vi "DevScripts_EnumToEnum-GLAttr.vi"() -> ()   [LabVIEW 2024]
uses:
  <vilib>/Utility/error.llb/Trim Whitespace One-Sided.vi
  SDL3/Video/GLAttr--enum.ctl
  SDL3/Video/Video.lvlib
panel:
  out "spreadsheet string":string
  out "Array":string[](array[string])
  in  "#Define list":string="    SDL_GL_RED_SIZE,                    /**< the minimum number of bits for the red channel of the color buffer; defaults to 3. */\n    SDL_GL_GREEN_SIZE,                  /**< the minimum number of bits for the green channel of the color buffer; defaults to 3. */\n    SDL_GL_BLUE_SIZE,                   /**< the minimum number of bits for the blue channel of the color buffer; defaults to 2. */\n    SDL_GL_ALPHA_SIZE,                  /**< the minimum number of bits for the alpha channel of the color buffer; defaults to 0. */\n    SDL_GL_BUFFER_SIZE,                 /**< the minimum number of bits for frame buffer size; defaults to 0. */\n    SDL_GL_DOUBLEBUFFER,                /**< whether the output is single or double buffered; defaults to double buffering on. */\n    SDL_GL_DEPTH_SIZE,                  /**< the minimum number of bits in the depth buffer; defaults to 16. */\n    SDL_GL_STENCIL_SIZE,                /**< the minimum number of bits in the stencil buffer; defaults to 0. */\n    SDL_GL_ACCUM_RED_SIZE,              /**< the minimum number of bits for the red channel of the accumulation buffer; defaults to 0. */\n    SDL_GL_ACCUM_GREEN_SIZE,            /**< the minimum number of bits for the green channel of the accumulation buffer; defaults to 0. */\n    SDL_GL_ACCUM_BLUE_SIZE,             /**< the minimum number of bits for the blue channel of the accumulation buffer; defaults to 0. */\n    SDL_GL_ACCUM_ALPHA_SIZE,            /**< the minimum number of bits for the alpha channel of the accumulation buffer; defaults to 0. */\n    SDL_GL_STEREO,                      /**< whether the output is stereo 3D; defaults to off. */\n    SDL_GL_MULTISAMPLEBUFFERS,          /**< the number of buffers used for multisample anti-aliasing; defaults to 0. */\n    SDL_GL_MULTISAMPLESAMPLES,          /**< the number of samples used around the current pixel used for multisample anti-aliasing. */\n    SDL_GL_ACCELERATED_VISUAL,          /**< set to 1 to require hardware acceleration, set to 0 to force software rendering; defaults to allow either. */\n    SDL_GL_RETAINED_BACKING,            /**< not used (deprecated). */\n    SDL_GL_CONTEXT_MAJOR_VERSION,       /**< OpenGL context major version. */\n    SDL_GL_CONTEXT_MINOR_VERSION,       /**< OpenGL context minor version. */\n    SDL_GL_CONTEXT_FLAGS,               /**< some combination of 0 or more of elements of the SDL_GLContextFlag enumeration; defaults to 0. */\n    SDL_GL_CONTEXT_PROFILE_MASK,        /**< type of GL context (Core, Compatibility, ES). See SDL_GLProfile; default value depends on platform. */\n    SDL_GL_SHARE_WITH_CURRENT_CONTEXT,  /**< OpenGL context sharing; defaults to 0. */\n    SDL_GL_FRAMEBUFFER_SRGB_CAPABLE,    /**< requests sRGB capable visual; defaults to 0. */\n    SDL_GL_CONTEXT_RELEASE_BEHAVIOR,    /**< sets context the release behavior. See SDL_GLContextReleaseFlag; defaults to FLUSH. */\n    SDL_GL_CONTEXT_RESET_NOTIFICATION,  /**< set context reset notification. See SDL_GLContextResetNotification; defaults to NO_NOTIFICATION. */\n    SDL_GL_CONTEXT_NO_ERROR,\n    SDL_GL_FLOATBUFFERS,\n    SDL_GL_EGL_PLATFORM"
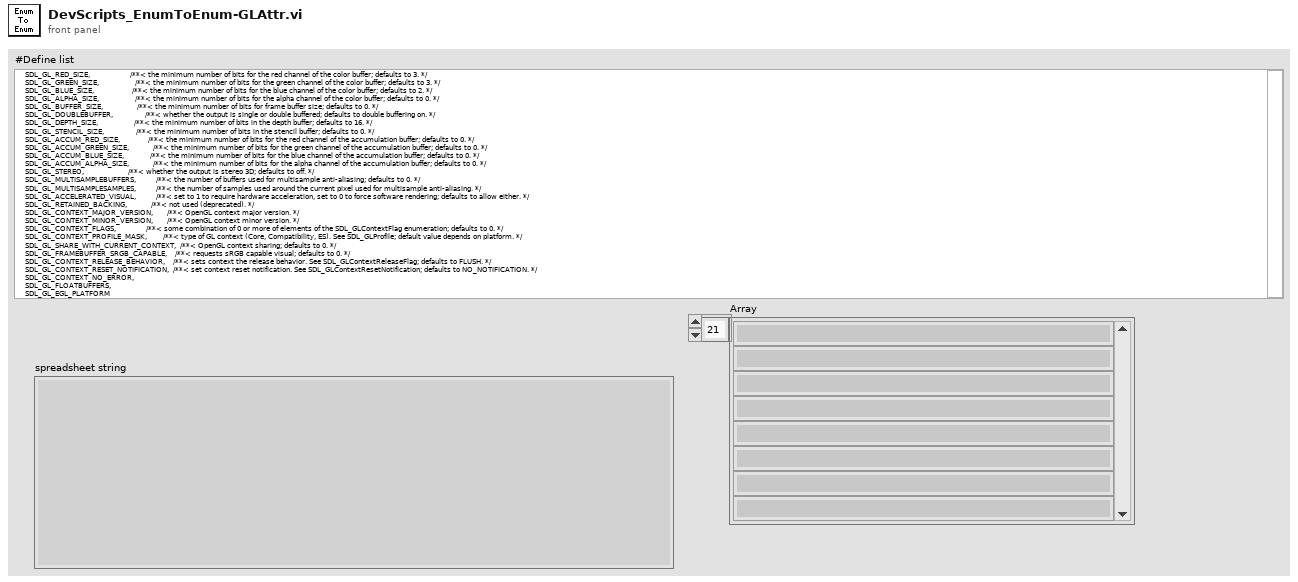
[diagram p1: front panel]
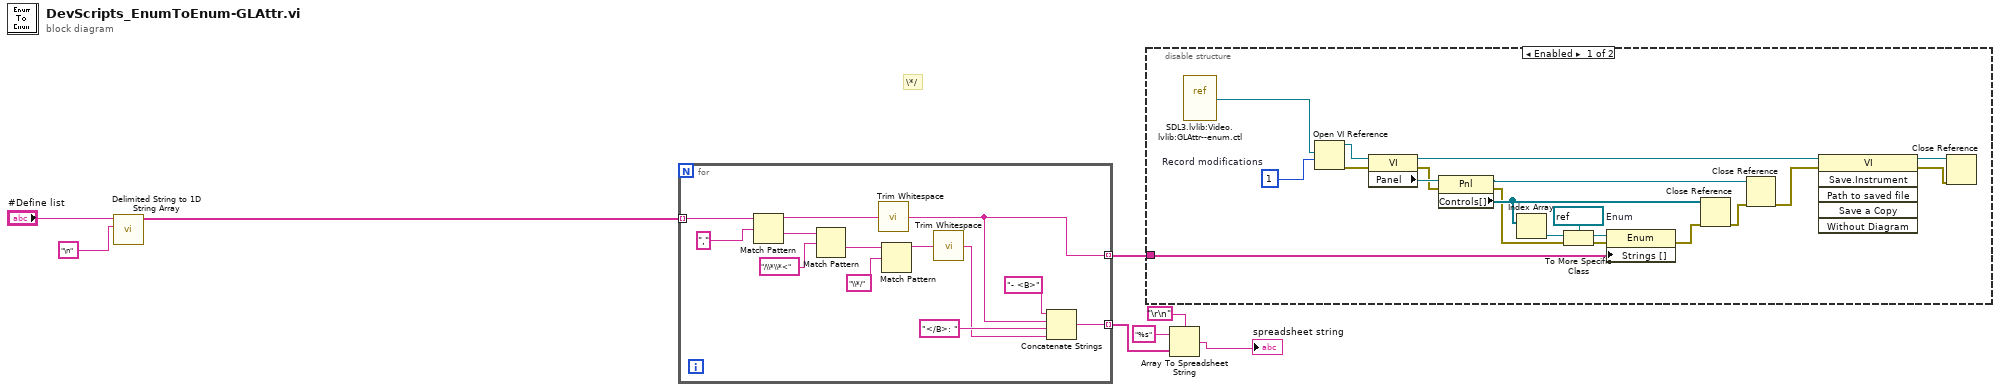
[diagram p0: block diagram]
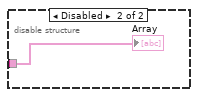
[diagram p2: hidden frame]
diagram:
  # "\\*/"
  n1 = call <vilib>:"Delimited String to 1D String Array.vi"("delimiter"="\n", "delimited string"="#Define list") -> ("string array"=w5:string[])  [unwired: 9 in]
  n2 = for {
    tunnel: w5 -> [w21] mode=indexing
    tunnel: [w12] -> w6 mode=indexing
    tunnel: [w9] -> w4 mode=indexing
    n3 = Match Pattern(string=w21, regular expression=",") -> (before substring=w19:string, after substring=w18:string)  [unwired: 1 in, 2 out]
    n4 = Match Pattern(string=w18, regular expression="/\\*\\*<") -> (after substring=w16:string)  [unwired: 1 in, 3 out]
    n5 = call <vilib>:"Trim Whitespace.vi"("string"=w19) -> ("trimmed string"=w12:string)  [unwired: 1 in]
    n6 = Match Pattern(string=w16, regular expression="\\*/") -> (before substring=w14:string)  [unwired: 1 in, 3 out]
    n7 = call <vilib>:"Trim Whitespace.vi"("string"=w14) -> ("trimmed string"=w10:string)  [unwired: 1 in]
    n8 = Concatenate Strings("- <B>" ("string"), w12, "</B>: " ("string"), w10) -> (w9:string)
  }
  n9 = disable-structure shown="Enabled" {
    disable-tunnel: w6 -> [w23 w42]
    frame Enabled {
      w33 = refnum<vi> refnum  # Enum
      w39 = 1  # Record modifications
      n10 = vi-ref "SDL3.lvlib:Video.lvlib:GLAttr--enum.ctl"() -> (w40:refnum<vi>)
      n11 = Open VI Reference(vi path=w40, options=w39) -> (vi reference=w38:refnum<vi>, error out=w41:errorcluster)  [unwired: 4 in]
      n12 = property class="VI"(reference=w38, error in=w41) -> (reference out=w28:refnum<vi>, error out=w36:errorcluster, "Panel"=w37:refnum<vi>)
      n13 = property class="Pnl"(reference=w37, error in=w36) -> (reference out=w35:refnum<vi>, error out=w26:errorcluster, "Controls[]"=w31:refnum<vi>[])
      n14 = Index Array(array=w31) -> (element=w32:refnum<vi>)  [unwired: 1 in]
      n15 = To More Specific Class(target class=w33, reference=w32, error in=w26) -> (specific class reference=w25:refnum<vi>, error out=w24:errorcluster)
      n16 = property class="Enum"(reference=w25, error in=w24, "Strings []"=w23) -> (error out=w22:errorcluster)  [unwired: 1 out]
      n17 = Close Reference(reference=w31, error in (no error)=w22) -> (error out=w30:errorcluster)
      n18 = Close Reference(reference=w35, error in (no error)=w30) -> (error out=w34:errorcluster)
      n19 = invoke class="VI" method="Save.Instrument"(reference=w28, error in=w34) -> (reference out=w27:refnum<vi>, error out=w29:errorcluster)  [unwired: 4 in, 4 out]
      n20 = Close Reference(reference=w27, error in (no error)=w29) -> ()  [unwired: 1 out]
    }
    frame Disabled {
      "Array" <- w42
    }
  }
  n21 = Array To Spreadsheet String(delimiter (Tab)="\r\n", array=w4, 3:"%s" ("format string")) -> (spreadsheet string=→"spreadsheet string":string)
